vi "PH_Cont-601k_PowerUnit.scr Charge.vi"(0 "VI in":refnum<vi>, 5 "error in (no error)":errorcluster) -> (14 "VI out":refnum<vi>, 19 "error out":errorcluster)   [LabVIEW 2014, in "PH_Cont-601k_PowerUnit.lvlib"]
uses:
  PH_Cont-601k_PowerUnit.lvlib
  PH_PowerUnit_BaseClass/PH_PowerUnit_BaseClass.SM States.ctl
  PH_Cont-601k_PSU/PH_Cont-601k_PSU.Readyness Device.ctl
  PH_PowerUnit_BaseClass/PH_PowerUnit_BaseClass.lvlib
  PH_Cont-601k_PSU/PH_Cont-601k_PSU.lvlib
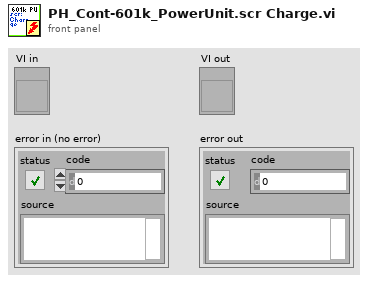
[diagram p1: front panel]
types:
  T1 = typedef "PH_Cont-601k_PSU.lvlib/PH_Cont-601k_PSU.Readyness Device.ctl" = enum32{"OFF", "CONNECTING", "CONNECTED", "OPERATING", "EOC", "ERROR"}
  T2 = typedef "PH_PowerUnit_BaseClass.lvlib/PH_PowerUnit_BaseClass.SM States.ctl" = enum16{".", "Stand by", "Switch PU on", "Configure", "Set Default Voltage", "Set STANDBY", "Set READY", "Wait for Shot Cmd", "Open Dump Rods", "Open Ross Relais", "Close Ross Relais", "Switch PSU on", "Switch PSU off", "Charge", "Switch GD Channel on", "Close Dump Rods", "Rods-TO", "RR-TO", "PSU-TO", "Trigger-TO"}
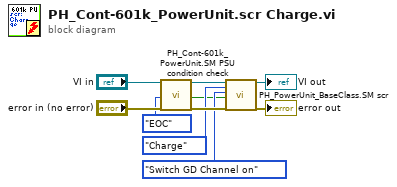
[diagram p0: block diagram]
diagram:
  n1 = call "PH_Cont-601k_PowerUnit.SM PSU condition check.vi"("VI in"="VI in", "Wanted Device Readyness (OPERATING)"=PH_Cont-601k_PSU.Readyness_Device."EOC" ("Wanted Device Readyness (Operating)"), "error in (no error)"="error in (no error)") -> ("VI out"=w8:refnum<vi>, "Condition fullfilled"=w2:bool, "error out"=w7:errorcluster)  [unwired: 14 in]
  n2 = call "PH_PowerUnit_BaseClass.SM scr.vi"("VI in"=w8, "Current SM State (condition)"=PH_PowerUnit_BaseClass.SM_States."Charge" ("SM State"), "Wanted SM State"=PH_PowerUnit_BaseClass.SM_States."Switch GD Channel on" ("SM State"), "Further change condition"=w2, "error in (no error)"=w7) -> ("VI out"=→"VI out":refnum<vi>, "error out"=→"error out":errorcluster)  [unwired: 13 in]
